vi "ConnectCamera.vi"(8 "error in (no error)":errorcluster, 11 "CameraTestingBL in":refnum<class "CameraTesting.lvclass">) -> (0 "error out":errorcluster, 3 "CameraTestingBL out":refnum<class "CameraTesting.lvclass">)   [LabVIEW 2020, in "CameraTesting.lvlib" / "CameraTesting.lvclass"]
doc: "Connect to Camera"
uses:
  CameraTesting.lvclass
  CameraTesting.lvclass/CameraTesting.ctl
  <vilib>/ActorFramework/Message Enqueuer/Message Enqueuer.lvclass/Message Enqueuer.ctl
  <vilib>/ActorFramework/Message Enqueuer/Enqueue.vi
  ICameraTestingUI/ICameraTestingUI Messages/ConnectCameraRslt Msg/ConnectCameraRslt Msg.lvclass
  C:/Program Files (x86)/National Instruments/LabVIEW 2020/vi.lib/ActorFramework/Message/Message.lvclass
  <vilib>/ActorFramework/Message Priority Queue/Priority Enqueue.vi
  Camera/ICamera/ICamera/ICamera.lvclass
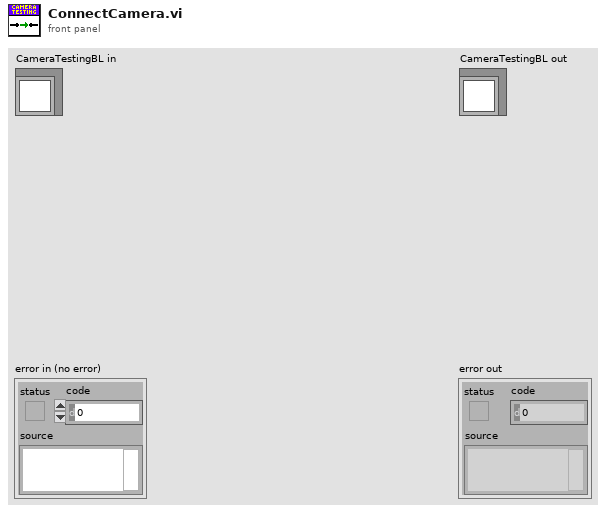
[diagram p1: front panel]
types:
  T1 = typedef "ICameraTesting.lvlib/ICameraTesting.lvclass/StatusUpdated.ctl" = refnum<user-event>
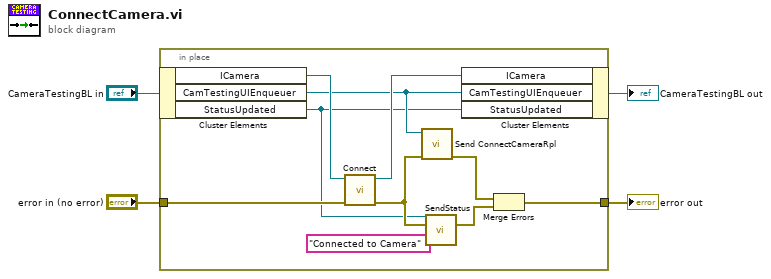
[diagram p0: block diagram]
diagram:
  n1 = in-place {
    in-place-border: "error in (no error)" -> [w14]
    in-place-border: [w5] -> w3
    n2 = in-place-cluster #1("CameraTestingBL in") -> ("ICamera"=w13:refnum<class "ICamera.lvclass">, "CamTestingUIEnqueuer"=w11:refnum<class "Message Enqueuer.lvclass">, "StatusUpdated"=w9:T1)
    n3 = call-dynamic "Connect.vi"("error in (no error)"=w14, "ICamera in"=w13) -> ("error out"=w10:errorcluster, "ICamera out"=w12:refnum<class "ICamera.lvclass">)  [unwired: 8 in]
    n4 = call "Send ConnectCameraRpl.vi"("error in (no error)"=w10, "Message Enqueuer"=w11) -> ("error out"=w7:errorcluster)  [unwired: 8 in, 1 out]
    n5 = call "SendStatus.vi"("StatusUsrEvn"=w9, "error in"=w10, "Text"="Connected to Camera") -> ("error out"=w6:errorcluster)  [unwired: 24 in]
    n6 = in-place-cluster #1("ICamera"=w12, "CamTestingUIEnqueuer"=w11, "StatusUpdated"=w9) -> (→"CameraTestingBL out":refnum<class "CameraTesting.lvclass">)
    n7 = Merge Errors(w7, w6) -> (w5:errorcluster)
  }
  "error out" <- w3
